vi "New Report.vi"(0 "window state (normal)":T2(ring)=enum."normal", 5 "display alerts? (F)":bool, 7 "report type":T1(ring), 9 "template (empty)":path, 11 "error in (no error)":errorcluster, 12 "machine name (empty)":string) -> (4 "report out":refnum<class "NI_report.lvclass">, 15 "error out":errorcluster)   [LabVIEW 2020, in "NI_report.lvclass"]
doc: "This VI is deprecated. Use the following VI instead:\n\nvi.lib\\Utility\\NIReport.llb\\Create Report.vi\n\nCreates a new report."
uses:
  <vilib>/Utility/NIReport.llb/NI_report.lvclass
  <vilib>/Utility/NIReport.llb/HTML/NI_HTML.lvclass
  e:/builds/penguin/labview/branches/2020/dev/dist/vi.lib/Utility/NIReport.llb/NI_report.lvclass
  <vilib>/Utility/NIReport.llb/Standard Report/NI_Standard Report.lvclass
  <vilib>/Utility/NIReport.llb/NI_ReportGenerationCore.lvlib
panel:
  # "This VI is deprecated. Use the following VI instead:\n\nvi.lib\\Utility\\NIReport.llb\\Create Report.vi"
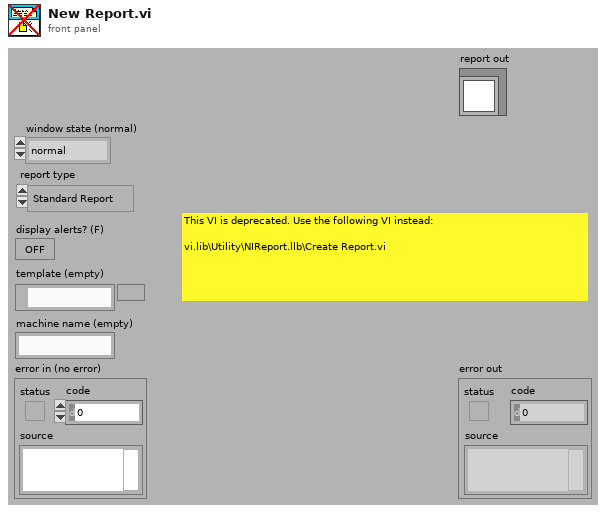
[diagram p1: front panel]
types:
  T1 = enum16{"Standard Report", "HTML", "Word", "Excel"}
  T2 = enum16{"maximized", "minimized", "normal", "no change"}
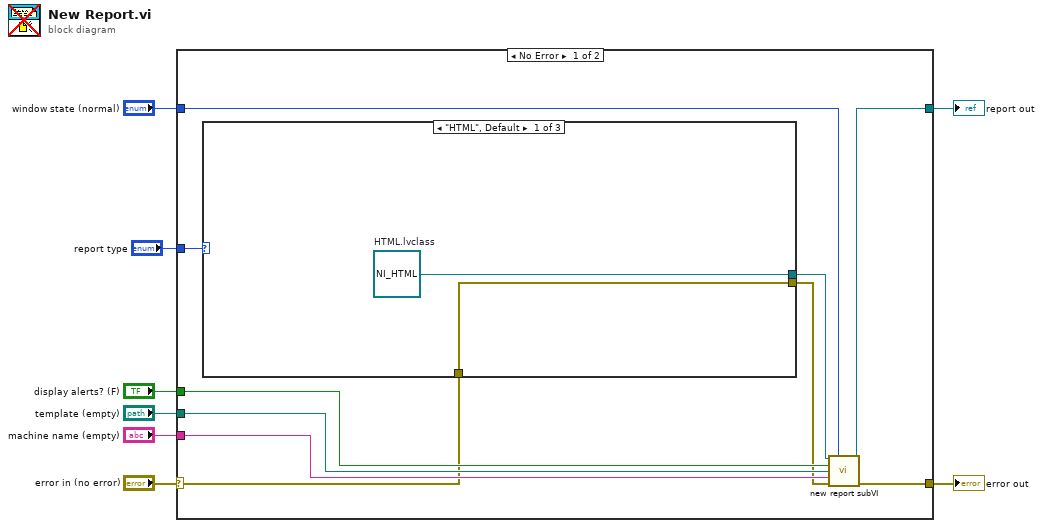
[diagram p0: block diagram]
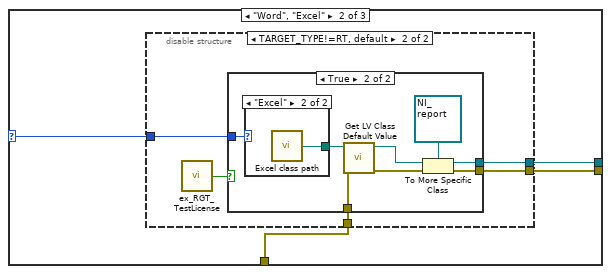
[diagram p2: hidden frame]
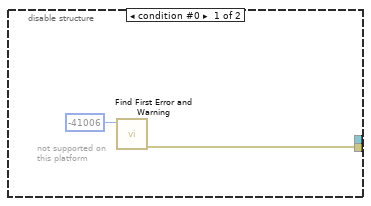
[diagram p3: hidden frame]
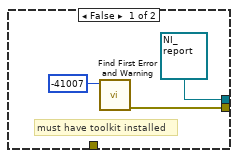
[diagram p4: hidden frame]
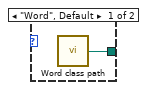
[diagram p5: hidden frame]
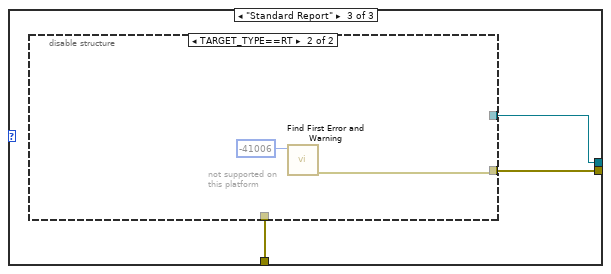
[diagram p6: hidden frame]
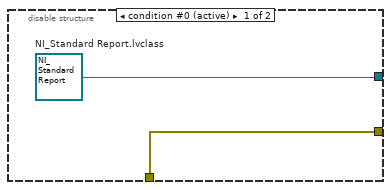
[diagram p7: hidden frame]
diagram:
  n1 = case shown="No Error" "error in (no error)" {
    selector: "error in (no error)" -> [w10 w52]
    tunnel: [w17 w52] -> w7
    tunnel: [w18 _] -> w6
    tunnel: "report type" -> [w12 _]
    tunnel: "template (empty)" -> [w16 _]
    tunnel: "machine name (empty)" -> [w15 _]
    tunnel: "display alerts? (F)" -> [w14 _]
    tunnel: "window state (normal)" -> [w13 _]
    frame No Error {
      n2 = case shown="\"HTML\", Default" w12 {
        selector: w12 -> [_ w22 _]
        tunnel: [w20 w24 w45] -> w11
        tunnel: [w19 w23 w46] -> w9
        tunnel: w10 -> [w19 w21 w47]
        frame "HTML", Default {
          w20 = refnum<class "NI_HTML.lvclass"> refnum  # HTML.lvclass
        }
        frame "Word", "Excel" {
          n3 = disable-structure shown="TARGET_TYPE!=RT, default" {
            disable-tunnel: [_ w29] -> w24
            disable-tunnel: [w25 w28] -> w23
            disable-tunnel: w22 -> [_ w30]
            disable-tunnel: w21 -> [_ w27]
            frame condition #0 {
              # "not supported on this platform"
              n4 = call <vilib>:"Find First Error and Warning.vi"("error code"=-41006) -> ("error out"=w25:errorcluster)  [unwired: 2 in, 4 out]
            }
            frame condition #1 (active) {
              n5 = call <vilib>:"ex_RGT_TestLicense.vi"() -> ("RGT license valid?"=w31:bool)  [unwired: 15 out]
              n6 = case shown="True" w31 {
                tunnel: [refnum<class "NI_report.lvclass"> refnum ("report out") w42] -> w29
                tunnel: [w33 w40] -> w28
                tunnel: w30 -> [_ w39]
                tunnel: w27 -> [_ w36]
                frame False {
                  # "must have toolkit installed"
                  n7 = call <vilib>:"Find First Error and Warning.vi"("error code"=-41007) -> ("error out"=w33:errorcluster)  [unwired: 2 in, 4 out]
                }
                frame True {
                  n8 = case shown="\"Excel\"" w39 {
                    tunnel: [w43 w44] -> w38
                    frame "Word", Default {
                      n9 = call <vilib>:"Word class path.vi"() -> ("Word class path"=w43:path)  [unwired: 15 out]
                    }
                    frame "Excel" {
                      n10 = call <vilib>:"Excel class path.vi"() -> ("Excel class path"=w44:path)  [unwired: 15 out]
                    }
                  }
                  n11 = call <vilib>:"Get LV Class Default Value.vi"("error in (no error)"=w36, "class path"=w38) -> ("error out"=w35:errorcluster, "object"=w37:refnum<class>)  [unwired: 8 out]
                  n12 = To More Specific Class(target class=refnum<class "NI_report.lvclass"> refnum ("report out"), reference=w37, error in=w35) -> (specific class reference=w42:refnum<class "NI_report.lvclass">, error out=w40:errorcluster)
                }
              }
            }
          }
        }
        frame "Standard Report" {
          n13 = disable-structure shown="TARGET_TYPE==RT" {
            disable-tunnel: w47 -> [w48 _]
            disable-tunnel: [w48 w50] -> w46
            disable-tunnel: [w49 _] -> w45
            frame condition #0 (active) {
              w49 = refnum<class "NI_Standard Report.lvclass"> refnum  # NI_Standard Report.lvclass
            }
            frame condition #1 {
              # "not supported on this platform"
              n14 = call <vilib>:"Find First Error and Warning.vi"("error code"=-41006) -> ("error out"=w50:errorcluster)  [unwired: 2 in, 4 out]
            }
          }
        }
      }
      n15 = call-dynamic "new report subVI.vi"("report in"=w11, "window state (normal)"=w13, "display alerts? (F)"=w14, "template (empty)"=w16, "machine name (empty)"=w15, "error in (no error)"=w9) -> ("report out"=w18:refnum<class "NI_report.lvclass">, "error out"=w17:errorcluster)  [unwired: 8 out]
    }
    frame Error {
    }
  }
  "error out" <- w7
  "report out" <- w6
